vi "Stop RUN.vi"(8 "error in (no error)":errorcluster, 11 "TCP Writer in":refnum<class "TCP Writer.lvclass">) -> (0 "error out":errorcluster, 3 "TCP Writer out":refnum<class "TCP Writer.lvclass">)   [LabVIEW 2026, in "TALOS.lvlib" / "TCP Writer.lvlib" / "TCP Writer.lvclass"]
uses:
  TCP Writer.lvclass
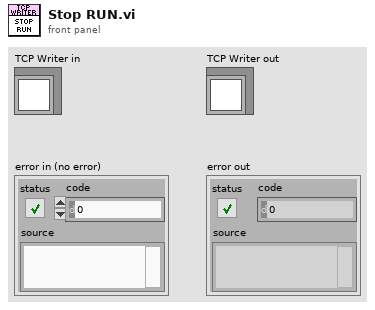
[diagram p1: front panel]
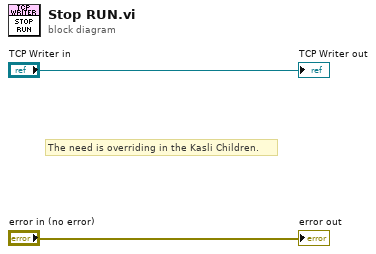
[diagram p0: block diagram]
diagram:
  # "The need is overriding in the Kasli Children."
  "error out" <- "error in (no error)"
  "TCP Writer out" <- "TCP Writer in"
